vi "Write FPGA Interface.vi"(8 "error in (no error)":errorcluster, 10 "FPGA Interface":refnum<class "FPGA Interface.lvclass">, 11 "1553 Test in":refnum<class "1553 Test.lvclass">) -> (0 "error out":errorcluster, 3 "1553 Test out":refnum<class "1553 Test.lvclass">)   [LabVIEW 2016, in "1553 Test.lvclass"]
uses:
  1553 Test.lvclass
  PPLs/FPGA Interface.lvlibp/FPGA Interface/FPGA Interface.lvclass
  1553 Test.lvclass/1553 Test.ctl
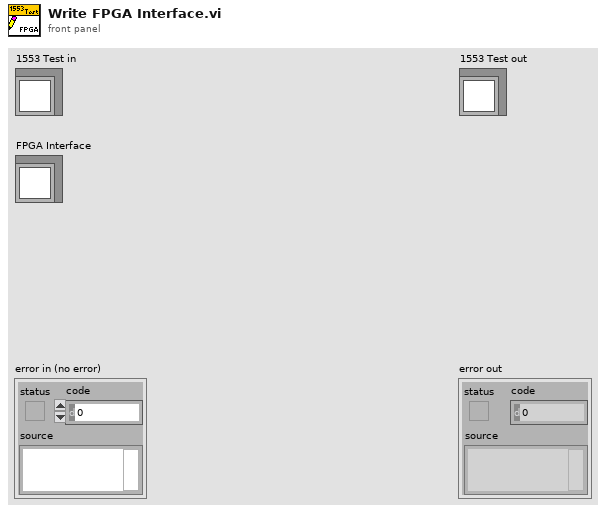
[diagram p1: front panel]
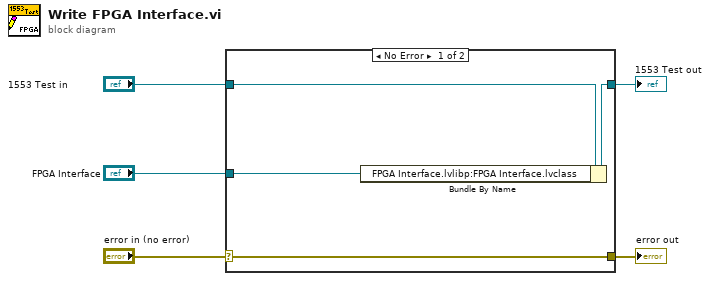
[diagram p0: block diagram]
diagram:
  n1 = case shown="No Error" "error in (no error)" {
    selector: "error in (no error)" -> [w9 w10]
    tunnel: [w9 w10] -> w4
    tunnel: [w7 w11] -> w2
    tunnel: "1553 Test in" -> [w8 w11]
    tunnel: "FPGA Interface" -> [w6 _]
    frame No Error {
      n2 = Bundle By Name(cluster=w8, "FPGA Interface.lvlibp:FPGA Interface.lvclass"=w6) -> (w7:refnum<class "1553 Test.lvclass">)
    }
    frame Error {
    }
  }
  "error out" <- w4
  "1553 Test out" <- w2
